vi "Calculate S Parameters.vi"(0 "Vector Path in":refnum<class "Vector Abstract Path.lvclass">, 11 "error in (no error)":errorcluster) -> (4 "Vector Path out":refnum<class "Vector Abstract Path.lvclass">, 6 "Frequencies":dbl[](array[numeric]), 8 "S Parameters out":cdb[][](array[numeric]), 15 "error out":errorcluster)   [LabVIEW 2023, in "RFFixtureCharact.Public.lvlib" / "Vector Abstract Path.lvclass"]
uses:
  Vector Abstract Path.lvclass
  Vector Abstract Path.lvclass/Vector Abstract Path.ctl
  Properties/Read Cal Standard Port.vi
  Instruments/Cal Standard/Cal Standard Base/Cal Standard Base.lvclass
  Instruments/Cal Standard/Cal Standard Factory/Cal Standard Factory.lvclass
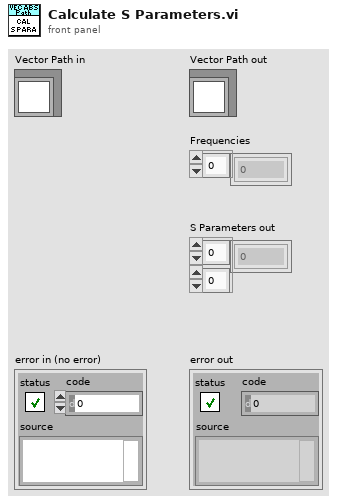
[diagram p1: front panel]
types:
  T1 = typedef "RFFixtureCharact.Instruments.lvlib/One-Port Charact Data.ctl" = cluster{"Standard Type":T2, "Frequencies":dbl[], "S11":cdb[]}
  T2 = typedef "RFFixtureCharact.Instruments.lvlib/Standard Type.ctl" = enum16{"Short", "Open", "Load", "PowerMeter", "None"}
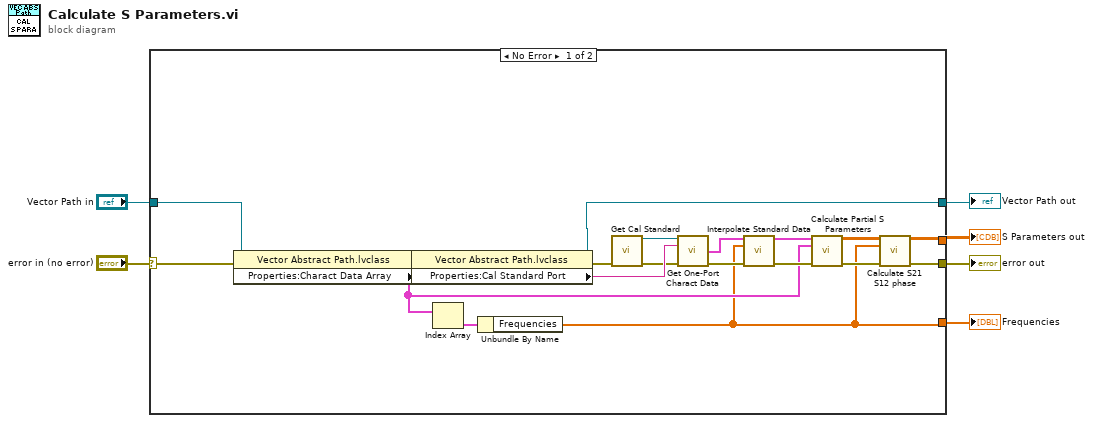
[diagram p0: block diagram]
diagram:
  n1 = case shown="No Error" "error in (no error)" {
    selector: "error in (no error)" -> [w7 w28]
    tunnel: [w8 w28] -> w4
    tunnel: "Vector Path in" -> [w15 w27]
    tunnel: [w9 w27] -> w3
    tunnel: [w11 _] -> w2
    tunnel: [w10 _] -> w1
    frame No Error {
      n2 = property class="Vector Abstract Path.lvclass"(reference=w15, error in=w7) -> (reference out=w13:refnum<class "Vector Abstract Path.lvclass">, error out=w12:errorcluster, "Properties:Charact Data Array"=w14:T1[])
      n3 = property class="Vector Abstract Path.lvclass"(reference=w13, error in=w12) -> (reference out=w9:refnum<class "Vector Abstract Path.lvclass">, error out=w19:errorcluster, "Properties:Cal Standard Port"=w26:string)
      n4 = Index Array(array=w14) -> (element=w16:T1)  [unwired: 1 in]
      n5 = Unbundle By Name(w16) -> ("Frequencies"=w11:dbl[])
      n6 = call "Get Cal Standard.vi"("error in (no error)"=w19) -> ("Cal Standard Base out"=w17:refnum<class "Cal Standard Base.lvclass">, "error out"=w18:errorcluster)  [unwired: 12 in, 1 out]
      n7 = call "Get One-Port Charact Data.vi"("Cal Standard in"=w17, "Port Name"=w26, "error in (no error)"=w18) -> ("One-Port Charact Data"=w20:T1[], "error out"=w21:errorcluster)  [unwired: 9 in, 2 out]
      n8 = call "Interpolate Standard Data.vi"("Standard Data"=w20, "Cal Frequencies"=w11, "error in (no error)"=w21) -> ("Interpolated Standard Data"=w24:T1[], "error out"=w25:errorcluster)  [unwired: 11 in]
      n9 = call "Calculate Partial S Parameters.vi"("Standard Data"=w24, "Result Data"=w14, "error in (no error)"=w25) -> ("S Parameters"=w22:cdb[][], "error out"=w23:errorcluster)  [unwired: 11 in]
      n10 = call "Calculate S21 S12 phase.vi"("S Parameters in"=w22, "Frequencies"=w11, "error in (no error)"=w23) -> ("S Parameters out"=w10:cdb[][], "error out"=w8:errorcluster)  [unwired: 11 in]
    }
    frame Error {
    }
  }
  "error out" <- w4
  "Vector Path out" <- w3
  "Frequencies" <- w2
  "S Parameters out" <- w1
